vi "GetDefaultCorr.vi"(8 "error in (no error)":errorcluster, 11 "AnalysisPluginsBase in":refnum<class "AnalysisPluginsBase.lvclass">) -> (0 "error out":errorcluster, 3 "AnalysisPluginsBase out":refnum<class "AnalysisPluginsBase.lvclass">)   [LabVIEW 2014, in "AnalysisPlugins.lvlib" / "AnalysisPluginsBase.lvclass"]
uses:
  AnalysisPluginsBase.lvclass
  <userlib>/NIST/BaseClasses/BasePlugin_class/BasePlugin.lvclass/BasePlugin.ctl
  AnalysisPluginsBase.lvclass/AnalysisPluginsBase.ctl
  <userlib>/NIST/BaseClasses/BasePlugin_class/Accessors/Read PluginIniFilePath.vi
  Accessors/Write DelayCorr.vi
  Accessors/Write MagCorr.vi
  <vilib>/Utility/error.llb/Error Cluster From Error Code.vi
  <vilib>/ErrorRing/Error Ring.xnode
  <vilib>/Utility/config.llb/NI_LVConfig.lvlib
panel:
  # "Gets the default correction values from the .ini file"
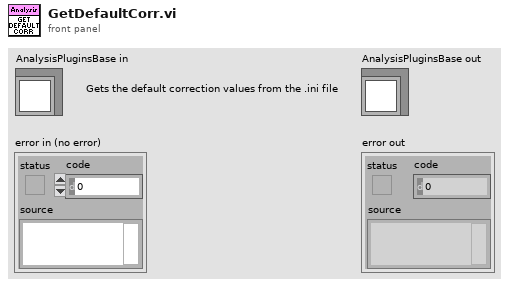
[diagram p1: front panel]
types:
  T1 = typedef "NI_LVConfig.lvlib/Config Data RefNum.ctl" = refnum<k1>
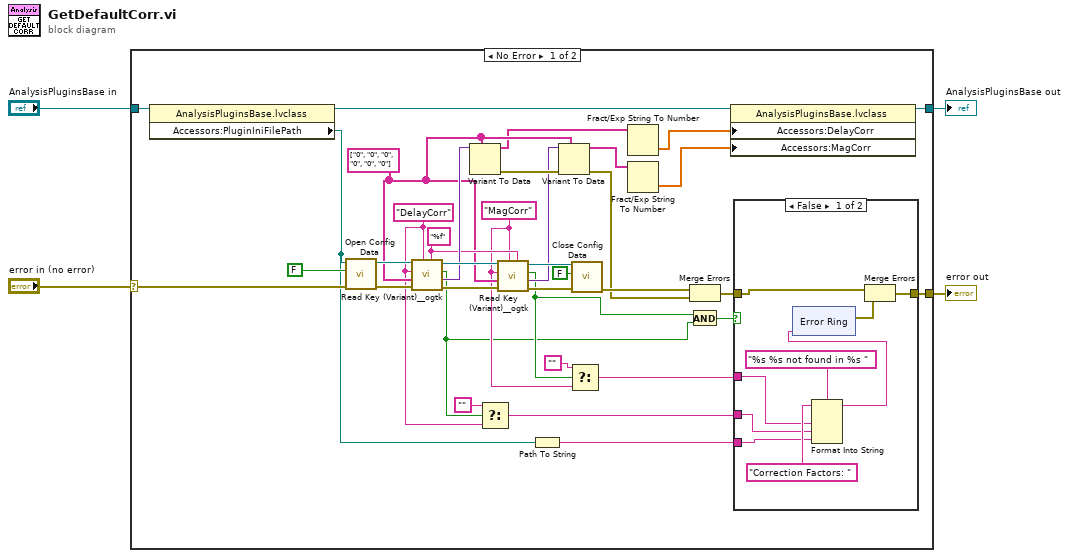
[diagram p0: block diagram]
diagram:
  n1 = case shown="No Error" "error in (no error)" {
    selector: "error in (no error)" -> [w38 w59]
    tunnel: [w16 w59] -> w3
    tunnel: [w25 w58] -> w1
    tunnel: "AnalysisPluginsBase in" -> [w40 w58]
    frame No Error {
      w23 = "%f" ("format string (%;%f)")
      w12 = "MagCorr" ("section (optional)")
      w14 = "DelayCorr" ("section (optional)")
      w22 = string[] ["0", "0", "0", "0", "0", "0"]
      n2 = property class="AnalysisPluginsBase.lvclass"(reference=w40) -> (reference out=w39:refnum<class "AnalysisPluginsBase.lvclass">, "Accessors:PluginIniFilePath"=w8:path)  [unwired: 1 in, 1 out]
      n3 = call <vilib>:"Open Config Data.vi"("error in (no error)"=w38, "create file if necessary (T)"=FALSE, "configuration file path"=w8) -> ("error out"=w36:errorcluster, "refnum"=w35:T1)  [unwired: 6 in, 1 out]
      n4 = call <userlib>:"Read Key (Variant)__ogtk.vi"("format string (%;%f)"=w23, "section"=w14, "error in (no error)"=w36, "type"=w22, "key (optional)"=w14, "refnum"=w35) -> ("error out"=w34:errorcluster, "key-value"=w29:variant, "found?"=w9:bool, "refnum out"=w33:T1)  [unwired: 2 in]
      n5 = Variant To Data(type=w22, Variant=w29) -> (data=w21:string[], error out=w28:errorcluster)  [unwired: 1 in]
      n6 = Select(t="", s=w9, f=w14) -> (s? t:f=w6:string)
      n7 = call <userlib>:"Read Key (Variant)__ogtk.vi"("format string (%;%f)"=w23, "section"=w12, "error in (no error)"=w34, "type"=w22, "key (optional)"=w12, "refnum"=w33) -> ("error out"=w32:errorcluster, "key-value"=w27:variant, "found?"=w10:bool, "refnum out"=w31:T1)  [unwired: 2 in]
      n8 = Path To String(path=w8) -> (string=w5:string)
      n9 = Variant To Data(error in=w28, type=w22, Variant=w27) -> (data=w20:string[], error out=w24:errorcluster)
      n10 = Select(t="", s=w10, f=w12) -> (s? t:f=w7:string)
      n11 = call <vilib>:"Close Config Data.vi"("error in (no error)"=w32, "write file if changed (T)"=FALSE, "refnum"=w31) -> ("error out"=w26:errorcluster)  [unwired: 7 in, 1 out]
      n12 = Fract/Exp String To Number(string=w21) -> (number=w19:dbl[])  [unwired: 3 in, 1 out]
      n13 = Fract/Exp String To Number(string=w20) -> (number=w18:dbl[])  [unwired: 3 in, 1 out]
      n14 = Merge Errors(w26, w24) -> (w17:errorcluster)
      n15 = And(x=w10, y=w9) -> (x .and. y?=w11:bool)
      n16 = property class="AnalysisPluginsBase.lvclass"(reference=w39, "Accessors:DelayCorr"=w19, "Accessors:MagCorr"=w18) -> (reference out=w25:refnum<class "AnalysisPluginsBase.lvclass">)  [unwired: 1 in, 1 out]
      n17 = case shown="False" w11 {
        tunnel: w17 -> [w42 w57]
        tunnel: [w43 w57] -> w16
        tunnel: w7 -> [w47 _]
        tunnel: w6 -> [w46 _]
        tunnel: w5 -> [w45 _]
        frame False {
          n18 = Format Into String(format string="%s %s not found in %s ", initial string="Correction Factors: ", w47, w46, w45) -> (resulting string=w44:string)  [unwired: 1 in, 1 out]
          n19 = xnode "Error Ring"("parameter 0"=w44) -> ("error out"=w41:errorcluster)
          n20 = Merge Errors(w42, w41) -> (w43:errorcluster)
        }
        frame True {
        }
      }
    }
    frame Error {
    }
  }
  "error out" <- w3
  "AnalysisPluginsBase out" <- w1
